vi "Get Test Case Item ID.vi"(8 "error in (no error)":errorcluster, 10 "Test Case":string, 11 "Icon Decorator In":refnum<class "Icon Decorator.lvclass">) -> (0 "error out":errorcluster, 2 "ObjectItem":T1)   [LabVIEW 2020, in "Icon Decorator.lvlib" / "Icon Decorator.lvclass"]
uses:
  Icon Decorator.lvclass
  <resource>/Framework/Providers/API/ItemRef.ctl
  Icon Decorator.lvclass/Icon Decorator.ctl
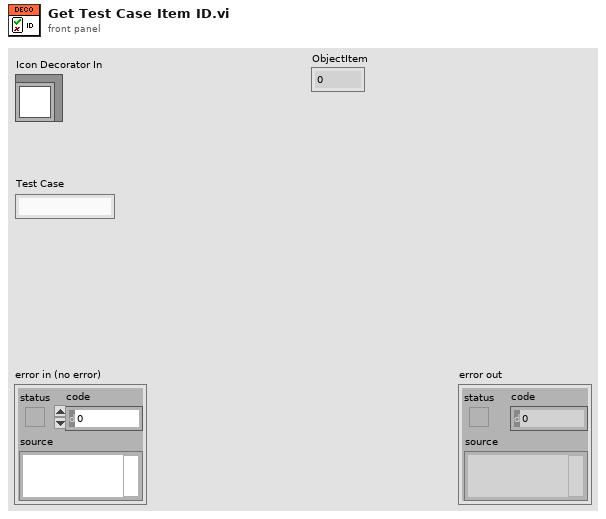
[diagram p1: front panel]
types:
  T1 = typedef "ItemRef.ctl" = u64
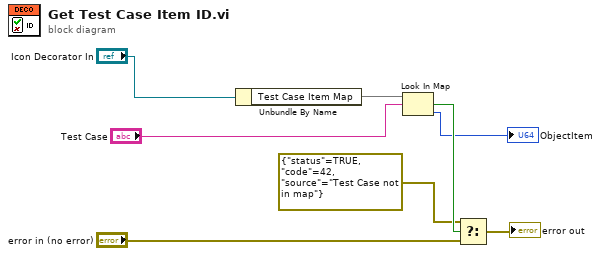
[diagram p0: block diagram]
diagram:
  n1 = Unbundle By Name("Icon Decorator In") -> ("Test Case Item Map"=w6:map{string, T1})
  n2 = Look In Map(map=w6, key="Test Case") -> (key not found?=w3:bool, value=→"ObjectItem":T1)  [unwired: 1 in]
  n3 = Select(t=errorcluster {"status"=TRUE, "code"=42, "source"="Test Case not in map"}, s=w3, f="error in (no error)") -> (s? t:f=→"error out":errorcluster)
